vi "Dispose Bitmap.vi"(8 "error in (no error)":errorcluster caption="错误输入（无错误）", 11 "Screen 输入":refnum<class "Screen.lvclass"> caption="DNL_LabVIEW Object in") -> (0 "error out":errorcluster caption="错误输出", 3 "Screen 输出":refnum<class "Screen.lvclass"> caption="DNL_LabVIEW Object out")   [LabVIEW 2011, in "Screen.lvclass"]
uses:
  Screen.lvclass
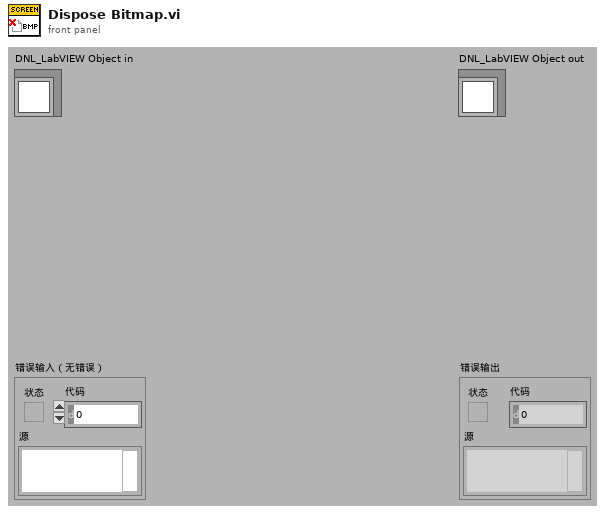
[diagram p1: front panel]
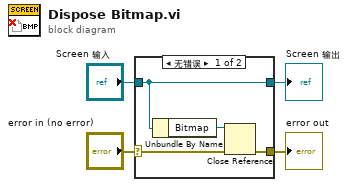
[diagram p0: block diagram]
diagram:
  n1 = case shown="无错误" "error in (no error)" {
    selector: "error in (no error)" -> [w6 w10]
    tunnel: [w5 w10] -> w3
    tunnel: [w8 w9] -> w1
    tunnel: "Screen 输入" -> [w8 w9]
    frame No Error {
      n2 = Unbundle By Name(w8) -> ("Bitmap"=w7:refnum<k24>)
      n3 = Close Reference(reference=w7, error in (no error)=w6) -> (error out=w5:errorcluster)
    }
    frame Error {
    }
  }
  "error out" <- w3
  "Screen 输出" <- w1
